vi "Initialize (SubVI).vi"(8 "error in (no error)":errorcluster, 11 "VISA Refnum in":refnum<visa-resource-name>) -> (0 "error out":errorcluster, 3 "VISA Refnum out":refnum<visa-resource-name>)   [LabVIEW 2021]
uses:
  8891b3a5-fc0c-455e-9730-2d727ea91fb9.vi
  5b16c787-849e-404d-86ee-f86a466d8160.vi
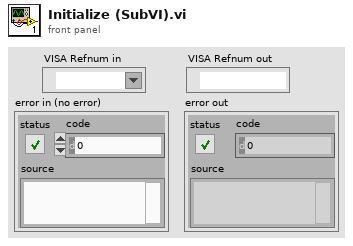
[diagram p1: front panel]
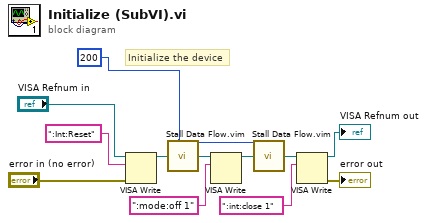
[diagram p0: block diagram]
diagram:
  w11 = u32 200 ("milliseconds to wait")
  # "Initialize the device"
  n1 = VISA Write(VISA resource name="VISA Refnum in", write buffer=":Int:Reset", error in (no error)="error in (no error)") -> (VISA resource name out=w8:refnum<visa-resource-name>)  [unwired: 2 out]
  n2 = call "Stall Data Flow.vim"("value in"=w8, "milliseconds to wait"=w11) -> ("value out"=w7:refnum<visa-resource-name>)  [unwired: 1 out]
  n3 = VISA Write(VISA resource name=w7, write buffer=":mode:off 1") -> (VISA resource name out=w9:refnum<visa-resource-name>)  [unwired: 1 in, 2 out]
  n4 = call "Stall Data Flow.vim"("value in"=w9, "milliseconds to wait"=w11) -> ("value out"=w10:refnum<visa-resource-name>)  [unwired: 1 out]
  n5 = VISA Write(VISA resource name=w10, write buffer=":int:close 1") -> (VISA resource name out=→"VISA Refnum out":refnum<visa-resource-name>, error out=→"error out":errorcluster)  [unwired: 1 in, 1 out]
